vi "Generate Random String.vi"(10 "String Length (32)":u32, 11 "RandomStringGenerator":refnum<class "RandomStringGenerator.lvclass">) -> (2 "Random String":string)   [LabVIEW 2014, in "RandomStringGenerator.lvclass"]
uses:
  RandomStringGenerator.lvclass
  RandomStringGenerator.lvclass/RandomStringGenerator.ctl
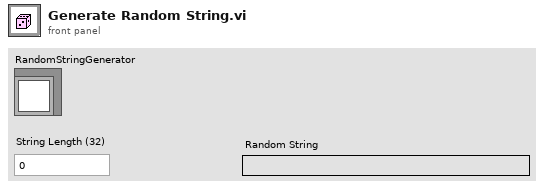
[diagram p1: front panel]
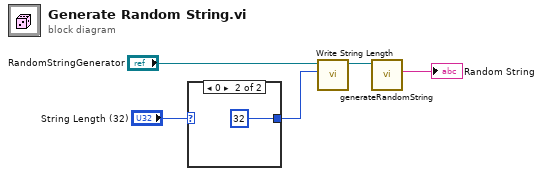
[diagram p0: block diagram]
diagram:
  n1 = case shown="0" "String Length (32)" {
    selector: "String Length (32)" -> [w6 _]
    tunnel: [w6 u32 32 ("String Length (32)")] -> w1
    frame Default {
    }
    frame 0 {
    }
  }
  n2 = call "Write String Length.vi"("String Length"=w1, "RandomStringGenerator in"="RandomStringGenerator") -> ("RandomStringGenerator out"=w3:refnum<class "RandomStringGenerator.lvclass">)  [unwired: 9 in]
  n3 = call-dynamic "generateRandomString.vi"("RandomStringGenerator in"=w3) -> ("Random String"=→"Random String":string)  [unwired: 9 in, 1 out]
